vi "Read targetConfigName.vi"(8 "error in (no error)":errorcluster, 11 "TargetConfiguration in":refnum<class "TargetConfiguration.lvclass">) -> (0 "error out":errorcluster, 2 "targetConfigName":string, 3 "TargetConfiguration out":refnum<class "TargetConfiguration.lvclass">)   [LabVIEW 2014, in "TCSDataDefinitions.lvlib" / "TCSCommand.lvlib" / "TargetConfiguration.lvlib" / "TargetConfiguration.lvclass"]
uses:
  TargetConfiguration.lvclass
  TargetConfiguration.lvclass/TargetConfiguration.ctl
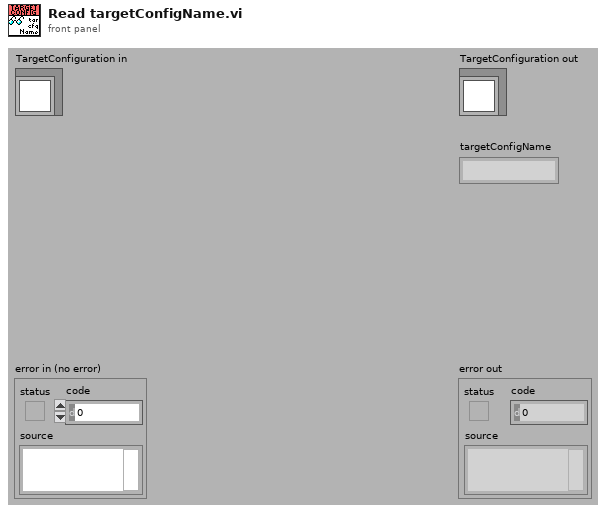
[diagram p1: front panel]
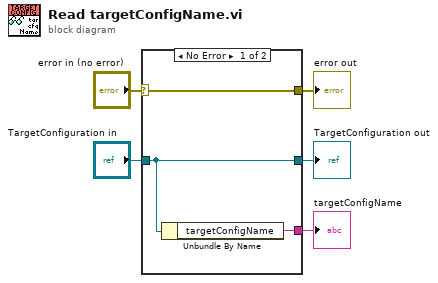
[diagram p0: block diagram]
diagram:
  n1 = case shown="No Error" "error in (no error)" {
    selector: "error in (no error)" -> [w8 w9]
    tunnel: [w8 w9] -> w4
    tunnel: [w7 w10] -> w2
    tunnel: "TargetConfiguration in" -> [w7 w10]
    tunnel: [w6 _] -> w1
    frame No Error {
      n2 = Unbundle By Name(w7) -> ("targetConfigName"=w6:string)
    }
    frame Error {
    }
  }
  "error out" <- w4
  "TargetConfiguration out" <- w2
  "targetConfigName" <- w1
